vi "Get PID Settings.vi"(0 "PI Far->Close":dbl[][](array[numeric]), 7 "SPzero":bool, 11 "Error":dbl) -> (4 "Slew":dbl, 6 "SlewIndex":dbl, 8 "Kp":dbl, 15 "Ki":dbl)   [LabVIEW 2013]
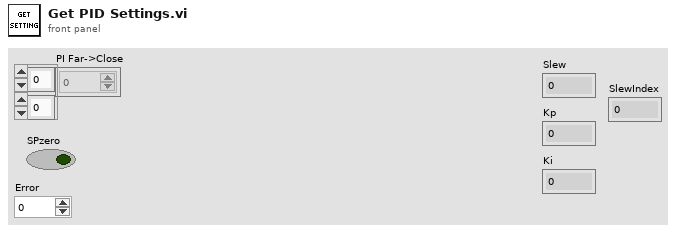
[diagram p1: front panel]
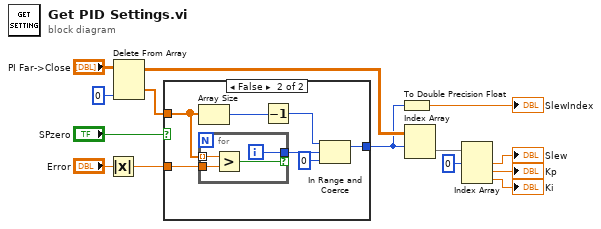
[diagram p0: block diagram]
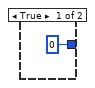
[diagram p2: hidden frame]
diagram:
  n1 = Absolute Value(x="Error") -> (abs(x)=w12:dbl)
  n2 = Delete From Array(array="PI Far->Close", index (col)=0 ("disabled index (col)")) -> (deleted portion=w11:dbl[], array with subset deleted=w10:dbl[][])  [unwired: 2 in]
  n3 = case shown="False" "SPzero" {
    tunnel: w12 -> [_ w22]
    tunnel: w11 -> [_ w20]
    tunnel: [0 ("lower limit") w17] -> w2
    frame True {
    }
    frame False {
      n4 = Array Size(array=w20) -> (size(s)=w19:i32)
      n5 = for {
        tunnel: w20 -> [w26] mode=indexing
        tunnel: w22 -> [w25]
        tunnel: [w24] -> w21 if=w23
        i -> [w24]
        n6 = Greater?(x=w26, y=w25) -> (0:w23:bool)
      }
      n7 = Decrement(x=w19) -> (x-1=w18:i32)
      n8 = In Range and Coerce(upper limit=w18, x=w21, lower limit=0) -> (coerced(x)=w17:i32)  [unwired: 1 out]
    }
  }
  n9 = To Double Precision Float(number=w2) -> (double precision float=→"SlewIndex":dbl)
  n10 = Index Array(array=w10, index (row)=w2) -> (element=w9:dbl[])  [unwired: 1 in]
  n11 = Index Array(array=w9, index #1=0 ("index")) -> (element #1=→"Slew":dbl, element #2=→"Kp":dbl, element #3=→"Ki":dbl)  [unwired: 2 in]
